vi "enteringState.vi"(8 "error in (no error)":errorcluster, 10 "State Data in":refnum<class "data.lvclass">, 11 "Target state in":refnum<class "state.lvclass">) -> (0 "error out":errorcluster, 2 "State Data out":refnum<class "data.lvclass">, 3 "Target state out":refnum<class "state.lvclass">)   [LabVIEW 2020, in "eos.lvlib" / "state.lvclass"]
uses:
  state.lvclass
  data/data.lvclass
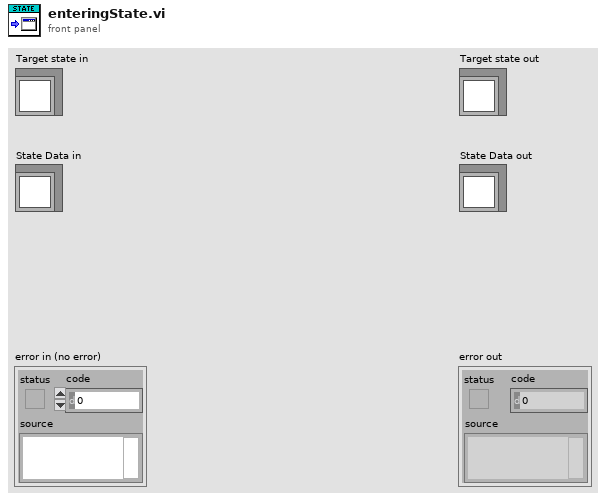
[diagram p1: front panel]
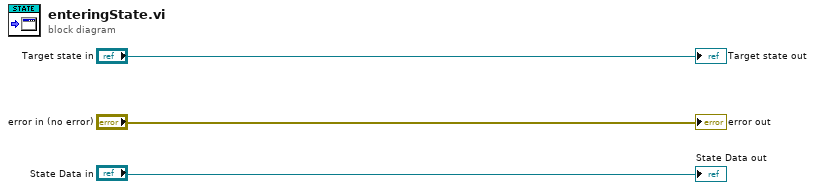
[diagram p0: block diagram]
diagram:
  "error out" <- "error in (no error)"
  "Target state out" <- "Target state in"
  "State Data out" <- "State Data in"
